vi "GetConnectionInfoFileName.vi"(8 "error in (no error)":errorcluster, 10 "hostname":string, 11 "upload path":path) -> (0 "error out":errorcluster, 1 "connInfo file":path, 2 "exists":bool, 3 "connection info":T1={"ClientName"="", "TransceiverHost"="", "TransceiverPort"=6342, "Password"=""})   [LabVIEW 2017, in "USBDrive.lvlib"]
uses:
  <vilib>/addons/InsightCM/Devices/Shared/Common/USBDrive/USBDrive.lvlib
  <vilib>/addons/InsightCM/MessageBus/Base/controls/ConnectionInfo.ctl
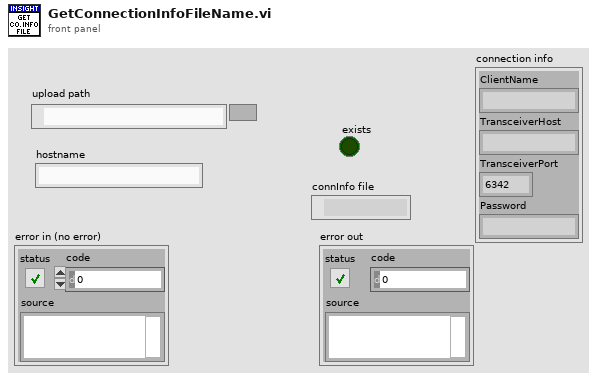
[diagram p1: front panel]
types:
  T1 = typedef "ConnectionInfo.ctl" = cluster{"ClientName":string, "TransceiverHost":string, "TransceiverPort":u16, "Password":string}
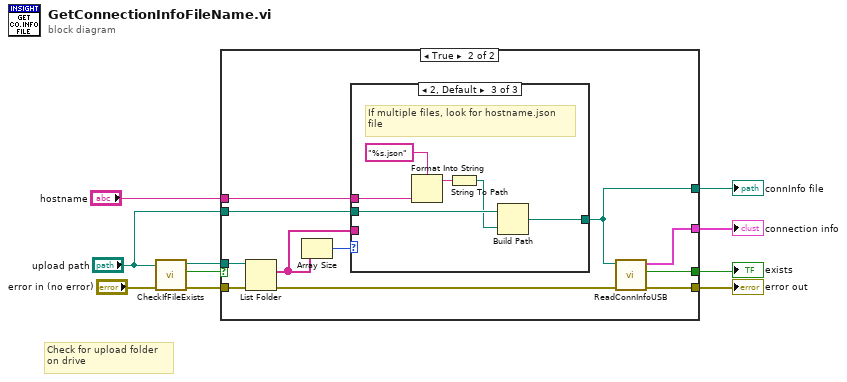
[diagram p0: block diagram]
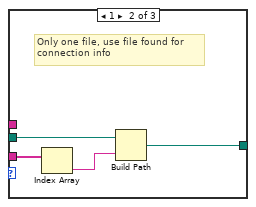
[diagram p4: hidden frame]
diagram:
  # "Check for upload folder\non drive"
  n1 = call <vilib>:"CheckIfFileExists.vi"("error in (no error)"="error in (no error)", "path"="upload path") -> ("error out"=w8:errorcluster, "file\\folder exists?"=w9:bool, "dup path"=w7:path)  [unwired: 7 in]
  n2 = case shown="True" w9 {
    tunnel: w8 -> [w11 w22]
    tunnel: w7 -> [_ w21]
    tunnel: "hostname" -> [_ w19]
    tunnel: [_ w15] -> w5
    tunnel: [w11 w14] -> w4
    tunnel: "upload path" -> [_ w17]
    tunnel: [_ w13] -> w2
    tunnel: [_ w12] -> w1
    frame False {
    }
    frame True {
      n3 = List Folder(path=w21, error in=w22) -> (filenames=w18:string[], error out=w16:errorcluster)  [unwired: 2 in, 2 out]
      n4 = Array Size(array=w18) -> (size(s)=w20:i32)
      n5 = case shown="2, Default" w20 {
        tunnel: w19 -> [_ _ w31]
        tunnel: [_ w23 w27] -> w12
        tunnel: w18 -> [_ w26 _]
        tunnel: w17 -> [_ w24 w29]
        frame 0 {
          # "No files found"
        }
        frame 1 {
          # "Only one file, use file found for \nconnection info"
          n6 = Index Array(array=w26) -> (element=w25:string)  [unwired: 1 in]
          n7 = Build Path(base path=w24, name or relative path=w25) -> (appended path=w23:path)
        }
        frame 2, Default {
          # "If multiple files, look for hostname.json\nfile"
          n8 = Format Into String(format string="%s.json", w31) -> (resulting string=w30:string)  [unwired: 2 in, 1 out]
          n9 = String To Path(string=w30) -> (path=w28:path)
          n10 = Build Path(base path=w29, name or relative path=w28) -> (appended path=w27:path)
        }
      }
      n11 = call <vilib>:"ReadConnInfoUSB.vi"("error in (no error)"=w16, "path"=w12) -> ("error out"=w14:errorcluster, "found"=w15:bool, "connection info"=w13:T1)  [unwired: 7 in]
    }
  }
  "exists" <- w5
  "error out" <- w4
  "connection info" <- w2
  "connInfo file" <- w1
